vi "Read Gantry Controller.vi"(8 "error in (no error)":errorcluster, 11 "Gantry in":refnum<class "Gantry.lvclass">) -> (0 "error out":errorcluster, 1 "Gantry Driver":T1, 2 "Aerotech Controller":variant, 3 "Gantry out":refnum<class "Gantry.lvclass">)   [LabVIEW 2024, in "Gantry.lvclass"]
uses:
  Gantry.lvclass
  Type Definitions/Gantry Driver.ctl
  Gantry.lvclass/Gantry.ctl
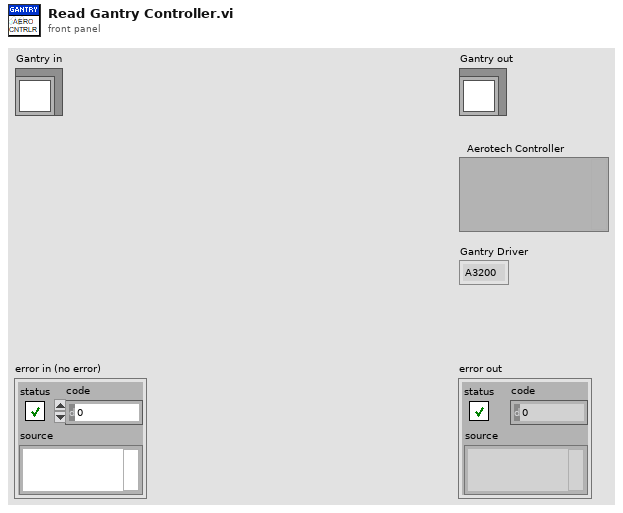
[diagram p1: front panel]
types:
  T1 = typedef "Gantry Driver.ctl" = enum16{"A3200", "AUTOMATION1", "VIRTUAL"}
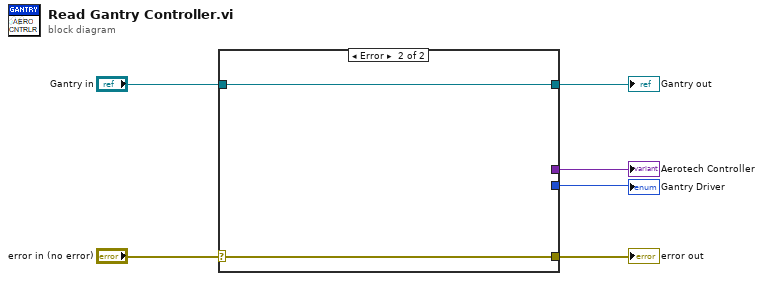
[diagram p0: block diagram]
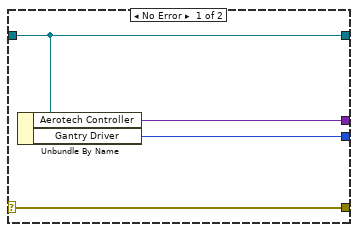
[diagram p2: hidden frame]
diagram:
  n1 = case shown="Error" "error in (no error)" {
    selector: "error in (no error)" -> [w10 w11]
    tunnel: [w10 w11] -> w5
    tunnel: [w9 w12] -> w3
    tunnel: "Gantry in" -> [w9 w12]
    tunnel: [w8 _] -> w2
    tunnel: [w7 _] -> w1
    frame No Error {
      n2 = Unbundle By Name(w9) -> ("Aerotech Controller"=w8:variant, "Gantry Driver"=w7:T1)
    }
    frame Error {
    }
  }
  "error out" <- w5
  "Gantry out" <- w3
  "Aerotech Controller" <- w2
  "Gantry Driver" <- w1
